vi "DDS_Close_Multiple_Boxes.vi"(8 "error in (no error)":errorcluster, 11 "DDS Settings":T1={"Enable DDS"=TRUE, "Array of DDS Boxes"=[]} {"Array of DDS Boxes"."Array of DDS Channels (4)"."Channel Parameters"."Ref Clock Rate [MHz]" min=0.0}) -> (0 "error out":errorcluster)   [LabVIEW 2014]
uses:
  DDS_Settings_Cluster.ctl
  DDS Library/Controls/DDS Box Array.ctl
  DDS Library/Controls/DDS Box Cluster.ctl
  DDS Library/Controls/DDS Box Device Reference.ctl
  <vilib>/ni845x/ni845x.llb/ni845xControl.ctl
  DDS Library/Controls/DDS Channel Array.ctl
  DDS Library/Controls/DDS Channel.ctl
  DDS Library/Controls/DDS Channel Parameters.ctl
  DDS Library/Controls/DDS RAM Destination.ctl
  DDS Library/Controls/DDS Profile Array.ctl
  DDS Library/Controls/DDS Profile.ctl
  DDS Library/Controls/DDS RAM Mode.ctl
  DDS Library/Controls/DDS RAM Timestep.ctl
  DDS Library/DDS.lvlib
  DDS.lvclass
panel:
  # "f/f/A"
  # "Mag"
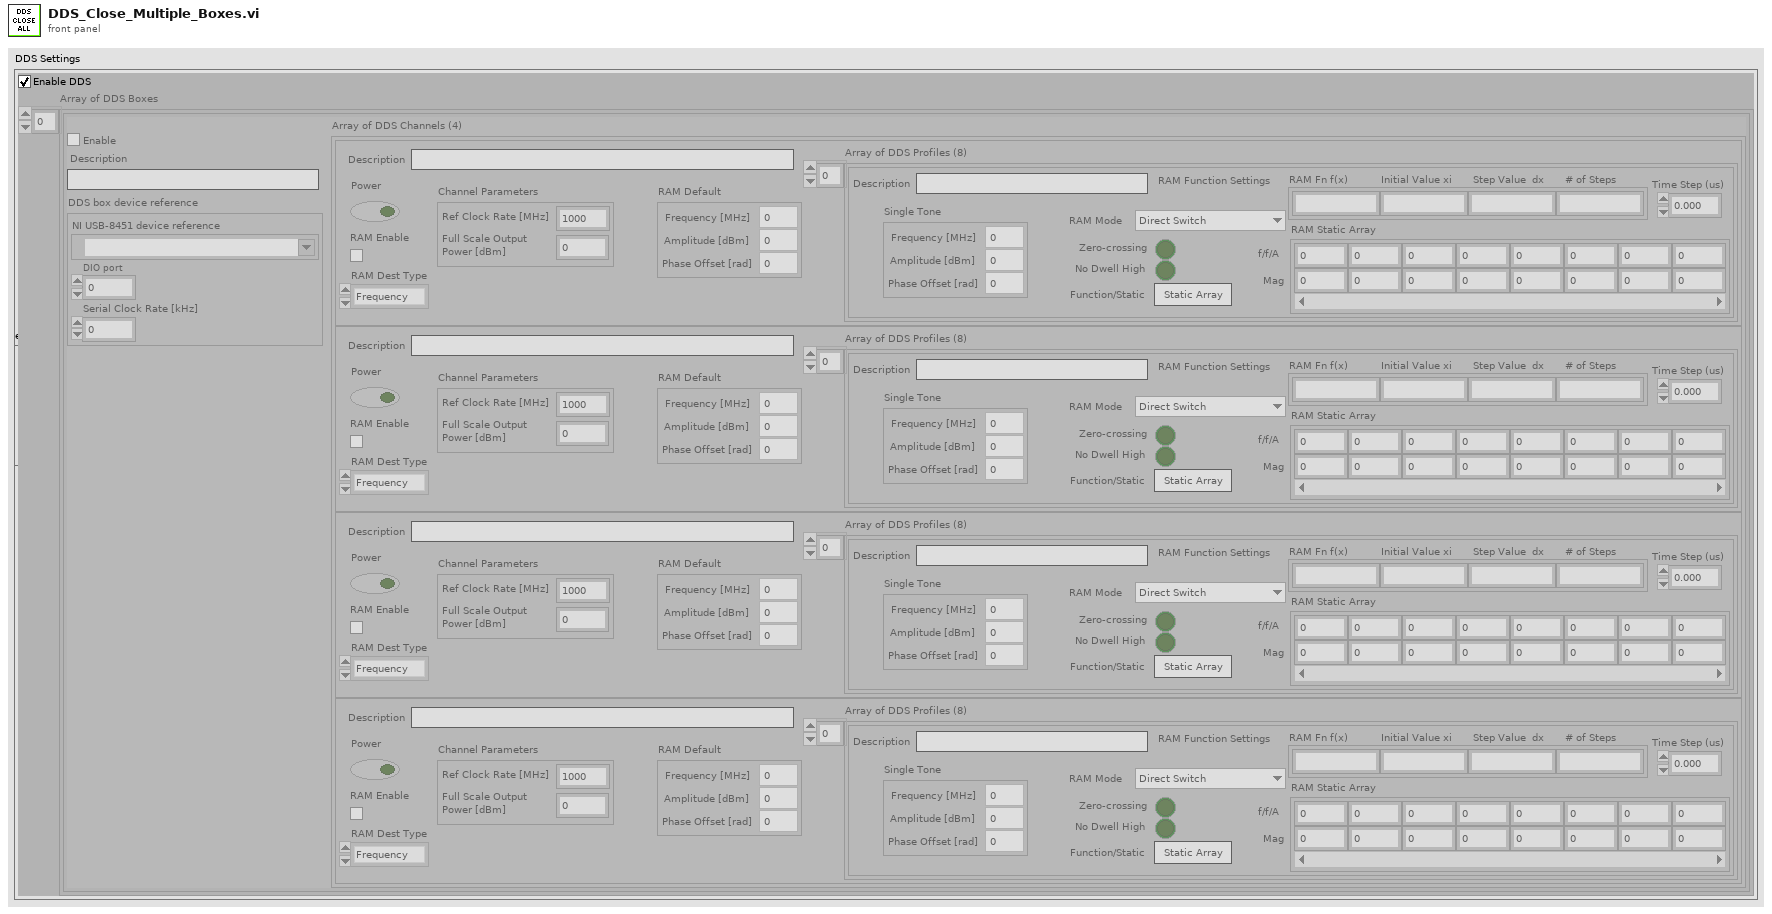
[diagram p1: front panel]
types:
  T1 = typedef "DDS.lvclass/DDS_Settings_Cluster.ctl" = cluster{"Enable DDS":bool, "Array of DDS Boxes":T2}
  T2 = typedef "DDS.lvlib/DDS Box Array.ctl" = T3[]
  T3 = typedef "DDS.lvlib/DDS Box Cluster.ctl" = cluster{"DDS box device reference":T4, "Array of DDS Channels (4)":T6, "Enable":bool, "Description":string}
  T4 = typedef "DDS.lvlib/DDS Box Device Reference.ctl" = cluster{"NI USB-8451 device reference":T5, "DIO port":u8, "Serial Clock Rate [kHz]":u16}
  T5 = typedef "ni845xControl.ctl" = refnum<k21>
  T6 = typedef "DDS.lvlib/DDS Channel Array.ctl" = T7[]
  T7 = typedef "DDS.lvlib/DDS Channel.ctl" = cluster{"Power":bool, "Channel Parameters":T8, "RAM Enable":bool, "RAM Dest Type":T9, "RAM Default":cluster{"Frequency [MHz]":dbl, "Amplitude [dBm]":dbl, "Phase Offset [rad]":dbl}, "Array of DDS Profiles (8)":T10, "Description":string}
  T8 = typedef "DDS.lvlib/DDS Channel Parameters.ctl" = cluster{"Ref Clock Rate [MHz]":dbl, "Full Scale Output\nPower [dBm]":dbl}
  T9 = typedef "DDS.lvlib/DDS RAM Destination.ctl" = enum16{"Frequency", "Phase", "Amplitude", "Polar"}
  T10 = typedef "DDS.lvlib/DDS Profile Array.ctl" = T11[]
  T11 = typedef "DDS.lvlib/DDS Profile.ctl" = cluster{"Single Tone":cluster{"Frequency [MHz]":dbl, "Amplitude [dBm]":dbl, "Phase Offset [rad]":dbl}, "RAM Mode ":T12, "Zero-crossing":bool, "No Dwell High":bool, "Function/Static":bool, "RAM Function Settings":string[], "RAM Static Array":dbl[][], "Description":string, "Time Step (us)":T13}
  T12 = typedef "DDS.lvlib/DDS RAM mode.ctl" = enum16{"Direct Switch", "Ramp Up", "Bidirectional Ramp", "Continuous Bidirectional Ramp", "Continuous Recirculate", "Direct Switch 2", "Direct Switch 3", "Direct Switch 4"}
  T13 = typedef "DDS.lvlib/DDS RAM Timestep.ctl" = dbl
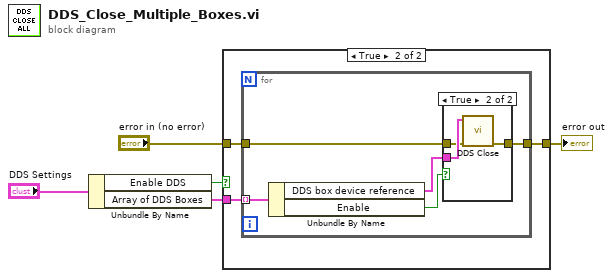
[diagram p0: block diagram]
diagram:
  n1 = Unbundle By Name("DDS Settings") -> ("Enable DDS"=w2:bool, "Array of DDS Boxes"=w1:T2)
  n2 = case shown="True" w2 {
    tunnel: "error in (no error)" -> [w6 w9]
    tunnel: [w6 w8] -> w4
    tunnel: w1 -> [_ w7]
    frame False {
    }
    frame True {
      n3 = for {
        tunnel: w9 -> [w14]
        tunnel: [w13] -> w8
        tunnel: w7 -> [w12] mode=indexing
        n4 = Unbundle By Name(w12) -> ("DDS box device reference"=w11:T4, "Enable"=w10:bool)
        n5 = case shown="True" w10 {
          tunnel: w14 -> [w15 w16]
          tunnel: [w15 w18] -> w13
          tunnel: w11 -> [_ w17]
          frame False {
          }
          frame True {
            n6 = call "DDS Close.vi"("error in (no error)"=w16, "DDS ref in"=w17) -> ("error out"=w18:errorcluster)  [unwired: 9 in]
          }
        }
      }
    }
  }
  "error out" <- w4
